vi "main.vi"() -> ()   [LabVIEW 2023] (continued)
     09\t16\t00\t00\tFF\tFF\tB0\t01\r\n       146  18F108A7   00000004    8        F0\t00\t00\tFF\tFF\tFF\tFF\t3E\r\n       145  18F106A7   00000004    8        00\tF7\tFF\tFF\tFF\tFF\tFF\t73\r\n       145  0CF104A7   00000004    8        F0\t60\t22\tFC\tFF\tFF\tFF\t39\r\n       144  0CF103A7   00000004    8        17\t1F\t08\t60\tB1\t1F\t08\t39\r\n       172  1FFFFFFF   00000004    8        00\t00\tFF\tFF\tFF\tFF\tFF\tFF\r\n       163  0CF102A7   00000004    8        30\t75\tE0\t2E\t80\tFF\tFF\tFD\r\n       163  0CF101A7   00000004    8        68\t00\t97\tCC\t00\t15\t39\t22\r\n       162  1FFFFFFF   00000004    8        00\t00\tFF\tFF\tFF\tFF\tFF\tFF\r\n       152  1FFFFFFF   00000004    8        00\t20\tFF\tFF\tFF\tFF\tFF\tFF\r\n       148  1FFFFFFF   00000004    8        00\t00\tFF\tFF\tFF\tFF\tFF\tFF\r\n       147  18FEF117   00000004    8        F7\t97\tCC\tCF\tFF\tFF\tFF\tFF\r\n       147  18F121F0   00000004    8        09\t16\t00\t00\tFF\tFF\tB0\t01\r\n       146  18F108A7   00000004    8        F0\t00\t00\tFF\tFF\tFF\tFF\t3E\r\n       145  18F106A7   00000004    8        00\tF7\tFF\tFF\tFF\tFF\tFF\t73\r\n       145  0CF104A7   00000004    8        F0\t60\t22\tFC\tFF\tFF\tFF\t39\r\n       182  1FFFFFFF   00000004    8        00\t00\tFF\tFF\tFF\tFF\tFF\tFF\r\n       172  1FFFFFFF   00000004    8        00\t00\tFF\tFF\tFF\tFF\tFF\tFF\r\n       163  0CF102A7   00000004    8        30\t75\tE0\t2E\t80\tFF\tFF\tFD\r\n       163  0CF101A7   00000004    8        68\t00\t97\tCC\t00\t15\t39\t22\r\n       162  1FFFFFFF   00000004    8        00\t00\tFF\tFF\tFF\tFF\tFF\tFF\r\n       152  1FFFFFFF   00000004    8        00\t20\tFF\tFF\tFF\tFF\tFF\tFF\r\n       148  1FFFFFFF   00000004    8        00\t00\tFF\tFF\tFF\tFF\tFF\tFF\r\n       147  18FEF117   00000004    8        F7\t97\tCC\tCF\tFF\tFF\tFF\tFF\r\n       147  18F121F0   00000004    8        09\t16\t00\t00\tFF\tFF\tB0\t01\r\n       146  18F108A7   00000004    8        F0\t00\t00\tFF\tFF\tFF\tFF\t3E\r\n       145  18F106A7   00000004    8        00\tF7\tFF\tFF\tFF\tFF\tFF\t73\r\n       183  0CF101A7   00000004    8        68\t00\t97\tCC\t00\t15\t39\t23\r\n       182  1FFFFFFF   00000004    8        00\t00\tFF\tFF\tFF\tFF\tFF\tFF\r\n       172  1FFFFFFF   00000004    8        00\t00\tFF\tFF\tFF\tFF\tFF\tFF\r\n       163  0CF102A7   00000004    8        30\t75\tE0\t2E\t80\tFF\tFF\tFD\r\n       163  0CF101A7   00000004    8        68\t00\t97\tCC\t00\t15\t39\t22\r\n       162  1FFFFFFF   00000004    8        00\t00\tFF\tFF\tFF\tFF\tFF\tFF\r\n       152  1FFFFFFF   00000004    8        00\t20\tFF\tFF\tFF\tFF\tFF\tFF\r\n       148  1FFFFFFF   00000004    8        00\t00\tFF\tFF\tFF\tFF\tFF\tFF\r\n       147  18FEF117   00000004    8        F7\t97\tCC\tCF\tFF\tFF\tFF\tFF\r\n       147  18F121F0   00000004    8        09\t16\t00\t00\tFF\tFF\tB0\t01\r\n       146  18F108A7   00000004    8        F0\t00\t00\tFF\tFF\tFF\tFF\t3E\r\n       183  0CF102A7   00000004    8        30\t75\tE0\t2E\t80\tFF\tFF\tFD\r\n       183  0CF101A7   00000004    8        68\t00\t97\tCC\t00\t15\t39\t23\r\n       182  1FFFFFFF   00000004    8        00\t00\tFF\tFF\tFF\tFF\tFF\tFF\r\n       172  1FFFFFFF   00000004    8        00\t00\tFF\tFF\tFF\tFF\tFF\tFF\r\n       163  0CF102A7   00000004    8        30\t75\tE0\t2E\t80\tFF\tFF\tFD\r\n       163  0CF101A7   00000004    8        68\t00\t97\tCC\t00\t15\t39\t22\r\n       162  1FFFFFFF   00000004    8        00\t00\tFF\tFF\tFF\tFF\tFF\tFF\r\n       152  1FFFFFFF   00000004    8        00\t20\tFF\tFF\tFF\tFF\tFF\tFF\r\n       148  1FFFFFFF   00000004    8        00\t00\tFF\tFF\tFF\tFF\tFF\tFF\r\n       147  18FEF117   00000004    8        F7\t97\tCC\tCF\tFF\tFF\tFF\tFF\r\n       147  18F121F0   00000004    8        09\t16\t00\t00\tFF\tFF\tB0\t01\r\n       192  1FFFFFFF   00000004    8        00\t00\tFF\tFF\tFF\tFF\tFF\tFF\r\n       183  0CF102A7   00000004    8        30\t75\tE0\t2E\t80\tFF\tFF\tFD\r\n       183  0CF101A7   00000004    8        68\t00\t97\tCC\t00\t15\t39\t23\r\n       182  1FFFFFFF   00000004    8        00\t00\tFF\tFF\tFF\tFF\tFF\tFF\r\n       172  1FFFFFFF   00000004    8        00\t00\tFF\tFF\tFF\tFF\tFF\tFF\r\n       163  0CF102A7   00000004    8        30\t75\tE0\t2E\t80\tFF\tFF\tFD\r\n       163  0CF101A7   00000004    8        68\t00\t97\tCC\t00\t15\t39\t22\r\n       162  1FFFFFFF   00000004    8        00\t00\tFF\tFF\tFF\tFF\tFF\tFF\r\n       152  1FFFFFFF   00000004    8        00\t20\tFF\tFF\tFF\tFF\tFF\tFF\r\n       148  1FFFFFFF   00000004    8        00\t00\tFF\tFF\tFF\tFF\tFF\tFF\r\n       147  18FEF117   00000004    8        F7\t97\tCC\tCF\tFF\tFF\tFF\tFF\r\n       193  18F106A7   00000004    8        00\tF7\tFF\tFF\tFF\tFF\tFF\t74\r\n       192  1FFFFFFF   00000004    8        00\t00\tFF\tFF\tFF\tFF\tFF\tFF\r\n       183  0CF102A7   00000004    8        30\t75\tE0\t2E\t80\tFF\tFF\tFD\r\n       183  0CF101A7   00000004    8        68\t00\t97\tCC\t00\t15\t39\t23\r\n       182  1FFFFFFF   00000004    8        00\t00\tFF\tFF\tFF\tFF\tFF\tFF\r\n       172  1FFFFFFF   00000004    8        00\t00\tFF\tFF\tFF\tFF\tFF\tFF\r\n       163  0CF102A7   00000004    8        30\t75\tE0\t2E\t80\tFF\tFF\tFD\r\n       163  0CF101A7   00000004    8        68\t00\t97\tCC\t00\t15\t39\t22\r\n       162  1FFFFFFF   00000004    8        00\t00\tFF\tFF\tFF\tFF\tFF\tFF\r\n       152  1FFFFFFF   00000004    8        00\t20\tFF\tFF\tFF\tFF\tFF\tFF\r\n       148  1FFFFFFF   00000004    8        00\t00\tFF\tFF\tFF\tFF\tFF\tFF\r\n       202  1FFFFFFF   00000004    8        00\t00\tFF\tFF\tFF\tFF\tFF\tFF\r\n       193  18F106A7   00000004    8        00\tF7\tFF\tFF\tFF\tFF\tFF\t74\r\n       192  1FFFFFFF   00000004    8        00\t00\tFF\tFF\tFF\tFF\tFF\tFF\r\n       183  0CF102A7   00000004    8        30\t75\tE0\t2E\t80\tFF\tFF\tFD\r\n       183  0CF101A7   00000004    8        68\t00\t97\tCC\t00\t15\t39\t23\r\n       182  1FFFFFFF   00000004    8        00\t00\tFF\tFF\tFF\tFF\tFF\tFF\r\n       172  1FFFFFFF   00000004    8        00\t00\tFF\tFF\tFF\tFF\tFF\tFF\r\n       163  0CF102A7   00000004    8        30\t75\tE0\t2E\t80\tFF\tFF\tFD\r\n       163  0CF101A7   00000004    8        68\t00\t97\tCC\t00\t15\t39\t22\r\n       162  1FFFFFFF   00000004    8        00\t00\tFF\tFF\tFF\tFF\tFF\tFF\r\n       152  1FFFFFFF   00000004    8        00\t20\tFF\tFF\tFF\tFF\tFF\tFF\r\n       203  0CF101A7   00000004    8        68\t00\t97\tCC\t00\t15\t39\t24\r\n       202  1FFFFFFF   00000004    8        00\t00\tFF\tFF\tFF\tFF\tFF\tFF\r\n       193  18F106A7   00000004    8        00\tF7\tFF\tFF\tFF\tFF\tFF\t74\r\n       192  1FFFFFFF   00000004    8        00\t00\tFF\tFF\tFF\tFF\tFF\tFF\r\n       183  0CF102A7   00000004    8        30\t75\tE0\t2E\t80\tFF\tFF\tFD\r\n       183  0CF101A7   00000004    8        68\t00\t97\tCC\t00\t15\t39\t23\r\n       182  1FFFFFFF   00000004    8        00\t00\tFF\tFF\tFF\tFF\tFF\tFF\r\n       172  1FFFFFFF   00000004    8        00\t00\tFF\tFF\tFF\tFF\tFF\tFF\r\n       163  0CF102A7   00000004    8        30\t75\tE0\t2E\t80\tFF\tFF\tFD\r\n       163  0CF101A7   00000004    8        68\t00\t97\tCC\t00\t15\t39\t22\r\n       162  1FFFFFFF   00000004    8        00\t00\tFF\tFF\tFF\tFF\tFF\tFF\r\n       203  0CF102A7   00000004    8        30\t75\tE0\t2E\t80\tFF\tFF\tFD\r\n       203  0CF101A7   00000004    8        68\t00\t97\tCC\t00\t15\t39\t24\r\n       202  1FFFFFFF   00000004    8        00\t00\tFF\tFF\tFF\tFF\tFF\tFF\r\n       193  18F106A7   00000004    8        00\tF7\tFF\tFF\tFF\tFF\tFF\t74\r\n       192  1FFFFFFF   00000004    8        00\t00\tFF\tFF\tFF\tFF\tFF\tFF\r\n       183  0CF102A7   00000004    8        30\t75\tE0\t2E\t80\tFF\tFF\tFD\r\n       183  0CF101A7   00000004    8        68\t00\t97\tCC\t00\t15\t39\t23\r\n       182  1FFFFFFF   00000004    8        00\t00\tFF\tFF\tFF\tFF\tFF\tFF\r\n       172  1FFFFFFF   00000004    8        00\t00\tFF\tFF\tFF\tFF\tFF\tFF\r\n       163  0CF102A7   00000004    8        30\t75\tE0\t2E\t80\tFF\tFF\tFD\r\n       163  0CF101A7   00000004    8        68\t00\t97\tCC\t00\t15\t39\t22\r\n       212  1FFFFFFF   00000004    8        00\t00\tFF\tFF\tFF\tFF\tFF\tFF\r\n       203  0CF102A7   00000004    8        30\t75\tE0\t2E\t80\tFF\tFF\tFD\r\n       203  0CF101A7   00000004    8        68\t00\t97\tCC\t00\t15\t39\t24\r\n       202  1FFFFFFF   00000004    8        00\t00\tFF\tFF\tFF\tFF\tFF\tFF\r\n       193  18F106A7   00000004    8        00\tF7\tFF\tFF\tFF\tFF\tFF\t74\r\n       192  1FFFFFFF   00000004    8        00\t00\tFF\tFF\tFF\tFF\tFF\tFF\r\n       183  0CF102A7   00000004    8        30\t75\tE0\t2E\t80\tFF\tFF\tFD\r\n       183  0CF101A7   00000004    8        68\t00\t97\tCC\t00\t15\t39\t23\r\n       182  1FFFFFFF   00000004    8        00\t00\tFF\tFF\tFF\tFF\tFF\tFF\r\n       172  1FFFFFFF   00000004    8        00\t00\tFF\tFF\tFF\tFF\tFF\tFF\r\n       163  0CF102A7   00000004    8        30\t75\tE0\t2E\t80\tFF\tFF\tFD\r\n       222  1FFFFFFF   00000004    8        00\t00\tFF\tFF\tFF\tFF\tFF\tFF\r\n       212  1FFFFFFF   00000004    8        00\t00\tFF\tFF\tFF\tFF\tFF\tFF\r\n       203  0CF102A7   00000004    8        30\t75\tE0\t2E\t80\tFF\tFF\tFD\r\n       203  0CF101A7   00000004    8        68\t00\t97\tCC\t00\t15\t39\t24\r\n       202  1FFFFFFF   00000004    8        00\t00\tFF\tFF\tFF\tFF\tFF\tFF\r\n       193  18F106A7   00000004    8        00\tF7\tFF\tFF\tFF\tFF\tFF\t74\r\n       192  1FFFFFFF   00000004    8        00\t00\tFF\tFF\tFF\tFF\tFF\tFF\r\n       183  0CF102A7   00000004    8        30\t75\tE0\t2E\t80\tFF\tFF\tFD\r\n       183  0CF101A7   00000004    8        68\t00\t97\tCC\t00\t15\t39\t23\r\n       182  1FFFFFFF   00000004    8        00\t00\tFF\tFF\tFF\tFF\tFF\tFF\r\n       172  1FFFFFFF   00000004    8        00\t00\tFF\tFF\tFF\tFF\tFF\tFF\r\n       223  0CF101A7   00000004    8        68\t00\t97\tCC\t00\t15\t39\t25\r\n       222  1FFFFFFF   00000004    8        00\t00\tFF\tFF\tFF\tFF\tFF\tFF\r\n       212  1FFFFFFF   00000004    8        00\t00\tFF\tFF\tFF\tFF\tFF\tFF\r\n       203  0CF102A7   00000004    8        30\t75\tE0\t2E\t80\tFF\tFF\tFD\r\n       203  0CF101A7   00000004    8        68\t00\t97\tCC\t00\t15\t39\t24\r\n       202  1FFFFFFF   00000004    8        00\t00\tFF\tFF\tFF\tFF\tFF\tFF\r\n       193  18F106A7   00000004    8        00\tF7\tFF\tFF\tFF\tFF\tFF\t74\r\n       192  1FFFFFFF   00000004    8        00\t00\tFF\tFF\tFF\tFF\tFF\tFF\r\n       183  0CF102A7   00000004    8        30\t75\tE0\t2E\t80\tFF\tFF\tFD\r\n       183  0CF101A7   00000004    8        68\t00\t97\tCC\t00\t15\t39\t23\r\n       182  1FFFFFFF   00000004    8        00\t00\tFF\tFF\tFF\tFF\tFF\tFF\r\n       223  0CF102A7   00000004    8        30\t75\tE0\t2E\t80\tFF\tFF\tFD\r\n       223  0CF101A7   00000004    8        68\t00\t97\tCC\t00\t15\t39\t25\r\n       222  1FFFFFFF   00000004    8        00\t00\tFF\tFF\tFF\tFF\tFF\tFF\r\n       212  1FFFFFFF   00000004    8        00\t00\tFF\tFF\tFF\tFF\tFF\tFF\r\n       203  0CF102A7   00000004    8        30\t75\tE0\t2E\t80\tFF\tFF\tFD\r\n       203  0CF101A7   00000004    8        68\t00\t97\tCC\t00\t15\t39\t24\r\n       202  1FFFFFFF   00000004    8        00\t00\tFF\tFF\tFF\tFF\tFF\tFF\r\n       193  18F106A7   00000004    8        00\tF7\tFF\tFF\tFF\tFF\tFF\t74\r\n       192  1FFFFFFF   00000004    8        00\t00\tFF\tFF\tFF\tFF\tFF\tFF\r\n       183  0CF102A7   00000004    8        30\t75\tE0\t2E\t80\tFF\tFF\tFD\r\n       183  0CF101A7   00000004    8        68\t00\t97\tCC\t00\t15\t39\t23\r\n       232  1FFFFFFF   00000004    8        00\t00\tFF\tFF\tFF\tFF\tFF\tFF\r\n       223  0CF102A7   00000004    8        30\t75\tE0\t2E\t80\tFF\tFF\tFD\r\n       223  0CF101A7   00000004    8        68\t00\t97\tCC\t00\t15\t39\t25\r\n       222  1FFFFFFF   00000004    8        00\t00\tFF\tFF\tFF\tFF\tFF\tFF\r\n       212  1FFFFFFF   00000004    8        00\t00\tFF\tFF\tFF\tFF\tFF\tFF\r\n       203  0CF102A7   00000004    8        30\t75\tE0\t2E\t80\tFF\tFF\tFD\r\n       203  0CF101A7   00000004    8        68\t00\t97\tCC\t00\t15\t39\t24\r\n       202  1FFFFFFF   00000004    8        00\t00\tFF\tFF\tFF\tFF\tFF\tFF\r\n       193  18F106A7   00000004    8        00\tF7\tFF\tFF\tFF\tFF\tFF\t74\r\n       192  1FFFFFFF   00000004    8        00\t00\tFF\tFF\tFF\tFF\tFF\tFF\r\n       183  0CF102A7   00000004    8        30\t75\tE0\t2E\t80\tFF\tFF\tFD\r\n       241  18F11FF0   00000004    8        FF\t3F\t90\t68\t88\t1B\t10\tAC\r\n       232  1FFFFFFF   00000004    8        00\t00\tFF\tFF\tFF\tFF\tFF\tFF\r\n       223  0CF102A7   00000004    8        30\t75\tE0\t2E\t80\tFF\tFF\tFD\r\n       223  0CF101A7   00000004    8        68\t00\t97\tCC\t00\t15\t39\t25\r\n       222  1FFFFFFF   00000004    8        00\t00\tFF\tFF\tFF\tFF\tFF\tFF\r\n       212  1FFFFFFF   00000004    8        00\t00\tFF\tFF\tFF\tFF\tFF\tFF\r\n       203  0CF102A7   00000004    8        30\t75\tE0\t2E\t80\tFF\tFF\tFD\r\n       203  0CF101A7   00000004    8        68\t00\t97\tCC\t00\t15\t39\t24\r\n       202  1FFFFFFF   00000004    8        00\t00\tFF\tFF\tFF\tFF\tFF\tFF\r\n       193  18F106A7   00000004    8        00\tF7\tFF\tFF\tFF\tFF\tFF\t74\r\n       192  1FFFFFFF   00000004    8        00\t00\tFF\tFF\tFF\tFF\tFF\tFF\r\n       242  18F120F0   00000004    8        2B\t75\t60\tB1\tB0\t01\tFF\tFF\r\n       241  18F11FF0   00000004    8        FF\t3F\t90\t68\t88\t1B\t10\tAC\r\n       232  1FFFFFFF   00000004    8        00\t00\tFF\tFF\tFF\tFF\tFF\tFF\r\n       223  0CF102A7   00000004    8        30\t75\tE0\t2E\t80\tFF\tFF\tFD\r\n       223  0CF101A7   00000004    8        68\t00\t97\tCC\t00\t15\t39\t25\r\n       222  1FFFFFFF   00000004    8        00\t00\tFF\tFF\tFF\tFF\tFF\tFF\r\n       212  1FFFFFFF   00000004    8        00\t00\tFF\tFF\tFF\tFF\tFF\tFF\r\n       203  0CF102A7   00000004    8        30\t75\tE0\t2E\t80\tFF\tFF\tFD\r\n       203  0CF101A7   00000004    8        68\t00\t97\tCC\t00\t15\t39\t24\r\n       202  1FFFFFFF   00000004    8        00\t00\tFF\tFF\tFF\tFF\tFF\tFF\r\n       193  18F106A7   00000004    8        00\tF7\tFF\tFF\tFF\tFF\tFF\t74\r\n       243  0CF101A7   00000004    8        68\t00\t97\tCC\t00\t15\t39\t26\r\n       242  18F120F0   00000004    8        2B\t75\t60\tB1\tB0\t01\tFF\tFF\r\n       241  18F11FF0   00000004    8        FF\t3F\t90\t68\t88\t1B\t10\tAC\r\n       232  1FFFFFFF   00000004    8        00\t00\tFF\tFF\tFF\tFF\tFF\tFF\r\n       223  0CF102A7   00000004    8        30\t75\tE0\t2E\t80\tFF\tFF\tFD\r\n       223  0CF101A7   00000004    8        68\t00\t97\tCC\t00\t15\t39\t25\r\n       222  1FFFFFFF   00000004    8        00\t00\tFF\tFF\tFF\tFF\tFF\tFF\r\n       212  1FFFFFFF   00000004    8        00\t00\tFF\tFF\tFF\tFF\tFF\tFF\r\n       203  0CF102A7   00000004    8        30\t75\tE0\t2E\t80\tFF\tFF\tFD\r\n       203  0CF101A7   00000004    8        68\t00\t97\tCC\t00\t15\t39\t24\r\n       202  1FFFFFFF   00000004    8        00\t00\tFF\tFF\tFF\tFF\tFF\tFF\r\n       243  0C3C4D4A   00000004    8        BE\tFF\tFF\t7F\t18\tFF\tFF\t3A\r\n       243  0CF101A7   00000004    8        68\t00\t97\tCC\t00\t15\t39\t26\r\n       242  18F120F0   00000004    8        2B\t75\t60\tB1\tB0\t01\tFF\tFF\r\n       241  18F11FF0   00000004    8        FF\t3F\t90\t68\t88\t1B\t10\tAC\r\n       232  1FFFFFFF   00000004    8        00\t00\tFF\tFF\tFF\tFF\tFF\tFF\r\n       223  0CF102A7   00000004    8        30\t75\tE0\t2E\t80\tFF\tFF\tFD\r\n       223  0CF101A7   00000004    8        68\t00\t97\tCC\t00\t15\t39\t25\r\n       222  1FFFFFFF   00000004    8        00\t00\tFF\tFF\tFF\tFF\tFF\tFF\r\n       212  1FFFFFFF   00000004    8        00\t00\tFF\tFF\tFF\tFF\tFF\tFF\r\n       203  0CF102A7   00000004    8        30\t75\tE0\t2E\t80\tFF\tFF\tFD\r\n       203  0CF101A7   00000004    8        68\t00\t97\tCC\t00\t15\t39\t24\r\n       244  0CF102A7   00000004    8        30\t75\tE0\t2E\t80\tFF\tFF\tFD\r\n       243  0C3C4D4A   00000004    8        BE\tFF\tFF\t7F\t18\tFF\tFF\t3A\r\n       243  0CF101A7   00000004    8        68\t00\t97\tCC\t00\t15\t39\t26\r\n       242  18F120F0   00000004    8        2B\t75\t60\tB1\tB0\t01\tFF\tFF\r\n       241  18F11FF0   00000004    8        FF\t3F\t90\t68\t88\t1B\t10\tAC\r\n       232  1FFFFFFF   00000004    8        00\t00\tFF\tFF\tFF\tFF\tFF\tFF\r\n       223  0CF102A7   00000004    8        30\t75\tE0\t2E\t80\tFF\tFF\tFD\r\n       223  0CF101A7   00000004    8        68\t00\t97\tCC\t00\t15\t39\t25\r\n       222  1FFFFFFF   00000004    8        00\t00\tFF\tFF\tFF\tFF\tFF\tFF\r\n       212  1FFFFFFF   00000004    8        00\t00\tFF\tFF\tFF\tFF\tFF\tFF\r\n       203  0CF102A7   00000004    8        30\t75\tE0\t2E\t80\tFF\tFF\tFD\r\n       244  0CF103A7   00000004    8        17\t1F\t08\t60\tB1\t1F\t08\t3A\r\n       244  0CF102A7   00000004    8        30\t75\tE0\t2E\t80\tFF\tFF\tFD\r\n       243  0C3C4D4A   00000004    8        BE\tFF\tFF\t7F\t18\tFF\tFF\t3A\r\n       243  0CF101A7   00000004    8        68\t00\t97\tCC\t00\t15\t39\t26\r\n       242  18F120F0   00000004    8        2B\t75\t60\tB1\tB0\t01\tFF\tFF\r\n       241  18F11FF0   00000004    8        FF\t3F\t90\t68\t88\t1B\t10\tAC\r\n       232  1FFFFFFF   00000004    8        00\t00\tFF\tFF\tFF\tFF\tFF\tFF\r\n       223  0CF102A7   00000004    8        30\t75\tE0\t2E\t80\tFF\tFF\tFD\r\n       223  0CF101A7   00000004    8        68\t00\t97\tCC\t00\t15\t39\t25\r\n       222  1FFFFFFF   00000004    8        00\t00\tFF\tFF\tFF\tFF\tFF\tFF\r\n       212  1FFFFFFF   00000004    8        00\t00\tFF\tFF\tFF\tFF\tFF\tFF\r\n       245  0CF104A7   00000004    8        F0\t60\t22\tFC\tFF\tFF\tFF\t3A\r\n       244  0CF103A7   00000004    8        17\t1F\t08\t60\tB1\t1F\t08\t3A\r\n       244  0CF102A7   00000004    8        30\t75\tE0\t2E\t80\tFF\tFF\tFD\r\n       243  0C3C4D4A   00000004    8        BE\tFF\tFF\t7F\t18\tFF\tFF\t3A\r\n       243  0CF101A7   00000004    8        68\t00\t97\tCC\t00\t15\t39\t26\r\n       242  18F120F0   00000004    8        2B\t75\t60\tB1\tB0\t01\tFF\tFF\r\n       241  18F11FF0   00000004    8        FF\t3F\t90\t68\t88\t1B\t10\tAC\r\n       232  1FFFFFFF   00000004    8        00\t00\tFF\tFF\tFF\tFF\tFF\tFF\r\n       223  0CF102A7   00000004    8        30\t75\tE0\t2E\t80\tFF\tFF\tFD\r\n       223  0CF101A7   00000004    8        68\t00\t97\tCC\t00\t15\t39\t25\r\n       222  1FFFFFFF   00000004    8        00\t00\tFF\tFF\tFF\tFF\tFF\tFF\r\n       246  18F106A7   00000004    8        00\tF7\tFF\tFF\tFF\tFF\tFF\t75\r\n       245  0CF104A7   00000004    8        F0\t60\t22\tFC\tFF\tFF\tFF\t3A\r\n       244  0CF103A7   00000004    8        17\t1F\t08\t60\tB1\t1F\t08\t3A\r\n       244  0CF102A7   00000004    8        30\t75\tE0\t2E\t80\tFF\tFF\tFD\r\n       243  0C3C4D4A   00000004    8        BE\tFF\tFF\t7F\t18\tFF\tFF\t3A\r\n       243  0CF101A7   00000004    8        68\t00\t97\tCC\t00\t15\t39\t26\r\n       242  18F120F0   00000004    8        2B\t75\t60\tB1\tB0\t01\tFF\tFF\r\n       241  18F11FF0   00000004    8        FF\t3F\t90\t68\t88\t1B\t10\tAC\r\n       232  1FFFFFFF   00000004    8        00\t00\tFF\tFF\tFF\tFF\tFF\tFF\r\n       223  0CF102A7   00000004    8        30\t75\tE0\t2E\t80\tFF\tFF\tFD\r\n       223  0CF101A7   00000004    8        68\t00\t97\tCC\t00\t15\t39\t25\r\n       246  18F121F0   00000004    8        09\t16\t00\t00\tFF\tFF\tB0\t01\r\n       246  18F106A7   00000004    8        00\tF7\tFF\tFF\tFF\tFF\tFF\t75\r\n       245  0CF104A7   00000004    8        F0\t60\t22\tFC\tFF\tFF\tFF\t3A\r\n       244  0CF103A7   00000004    8        17\t1F\t08\t60\tB1\t1F\t08\t3A\r\n       244  0CF102A7   00000004    8        30\t75\tE0\t2E\t80\tFF\tFF\tFD\r\n       243  0C3C4D4A   00000004    8        BE\tFF\tFF\t7F\t18\tFF\tFF\t3A\r\n       243  0CF101A7   00000004    8        68\t00\t97\tCC\t00\t15\t39\t26\r\n       242  18F120F0   00000004    8        2B\t75\t60\tB1\tB0\t01\tFF\tFF\r\n       241  18F11FF0   00000004    8        FF\t3F\t90\t68\t88\t1B\t10\tAC\r\n       232  1FFFFFFF   00000004    8        00\t00\tFF\tFF\tFF\tFF\tFF\tFF\r\n       223  0CF102A7   00000004    8        30\t75\tE0\t2E\t80\tFF\tFF\tFD\r\n       247  1FFFFFFF   00000004    8        00\t00\tFF\tFF\tFF\tFF\tFF\tFF\r\n       246  18F121F0   00000004    8        09\t16\t00\t00\tFF\tFF\tB0\t01\r\n       246  18F106A7   00000004    8        00\tF7\tFF\tFF\tFF\tFF\tFF\t75\r\n       245  0CF104A7   00000004    8        F0\t60\t22\tFC\tFF\tFF\tFF\t3A\r\n       244  0CF103A7   00000004    8        17\t1F\t08\t60\tB1\t1F\t08\t3A\r\n       244  0CF102A7   00000004    8        30\t75\tE0\t2E\t80\tFF\tFF\tFD\r\n       243  0C3C4D4A   00000004    8        BE\tFF\tFF\t7F\t18\tFF\tFF\t3A\r\n       243  0CF101A7   00000004    8        68\t00\t97\tCC\t00\t15\t39\t26\r\n       242  18F120F0   00000004    8        2B\t75\t60\tB1\tB0\t01\tFF\tFF\r\n       241  18F11FF0   00000004    8        FF\t3F\t90\t68\t88\t1B\t10\tAC\r\n       232  1FFFFFFF   00000004    8        00\t00\tFF\tFF\tFF\tFF\tFF\tFF\r\n       252  1FFFFFFF   00000004    8        00\t00\tFF\tFF\tFF\tFF\tFF\tFF\r\n       247  1FFFFFFF   00000004    8        00\t00\tFF\tFF\tFF\tFF\tFF\tFF\r\n       246  18F121F0   00000004    8        09\t16\t00\t00\tFF\tFF\tB0\t01\r\n       246  18F106A7   00000004    8        00\tF7\tFF\tFF\tFF\tFF\tFF\t75\r\n       245  0CF104A7   00000004    8        F0\t60\t22\tFC\tFF\tFF\tFF\t3A\r\n       244  0CF103A7   00000004    8        17\t1F\t08\t60\tB1\t1F\t08\t3A\r\n       244  0CF102A7   00000004    8        30\t75\tE0\t2E\t80\tFF\tFF\tFD\r\n       243  0C3C4D4A   00000004    8        BE\tFF\tFF\t7F\t18\tFF\tFF\t3A\r\n       243  0CF101A7   00000004    8        68\t00\t97\tCC\t00\t15\t39\t26\r\n       242  18F120F0   00000004    8        2B\t75\t60\tB1\tB0\t01\tFF\tFF\r\n       241  18F11FF0   00000004    8        FF\t3F\t90\t68\t88\t1B\t10\tAC\r\n       262  1FFFFFFF   00000004    8        00\t20\tFF\tFF\tFF\tFF\tFF\tFF\r\n       252  1FFFFFFF   00000004    8        00\t00\tFF\tFF\tFF\tFF\tFF\tFF\r\n       247  1FFFFFFF   00000004    8        00\t00\tFF\tFF\tFF\tFF\tFF\tFF\r\n       246  18F121F0   00000004    8        09\t16\t00\t00\tFF\tFF\tB0\t01\r\n       246  18F106A7   00000004    8        00\tF7\tFF\tFF\tFF\tFF\tFF\t75\r\n       245  0CF104A7   00000004    8        F0\t60\t22\tFC\tFF\tFF\tFF\t3A\r\n       244  0CF103A7   00000004    8        17\t1F\t08\t60\tB1\t1F\t08\t3A\r\n       244  0CF102A7   00000004    8        30\t75\tE0\t2E\t80\tFF\tFF\tFD\r\n       243  0C3C4D4A   00000004    8        BE\tFF\tFF\t7F\t18\tFF\tFF\t3A\r\n       243  0CF101A7   00000004    8        68\t00\t97\tCC\t00\t15\t39\t26\r\n       242  18F120F0   00000004    8        2B\t75\t60\tB1\tB0\t01\tFF\tFF\r\n       263  0CF101A7   00000004    8        68\t00\t97\tCC\t00\t15\t39\t27\r\n       262  1FFFFFFF   00000004    8        00\t20\tFF\tFF\tFF\tFF\tFF\tFF\r\n       252  1FFFFFFF   00000004    8        00\t00\tFF\tFF\tFF\tFF\tFF\tFF\r\n       247  1FFFFFFF   00000004    8        00\t00\tFF\tFF\tFF\tFF\tFF\tFF\r\n       246  18F121F0   00000004    8        09\t16\t00\t00\tFF\tFF\tB0\t01\r\n       246  18F106A7   00000004    8        00\tF7\tFF\tFF\tFF\tFF\tFF\t75\r\n       245  0CF104A7   00000004    8        F0\t60\t22\tFC\tFF\tFF\tFF\t3A\r\n       244  0CF103A7   00000004    8        17\t1F\t08\t60\tB1\t1F\t08\t3A\r\n       244  0CF102A7   00000004    8        30\t75\tE0\t2E\t80\tFF\tFF\tFD\r\n       243  0C3C4D4A   00000004    8        BE\tFF\tFF\t7F\t18\tFF\tFF\t3A\r\n       243  0CF101A7   00000004    8        68\t00\t97\tCC\t00\t15\t39\t26\r\n       263  0CF102A7   00000004    8        30\t75\tE0\t2E\t80\tFF\tFF\tFD\r\n       263  0CF101A7   00000004    8        68\t00\t97\tCC\t00\t15\t39\t27\r\n       262  1FFFFFFF   00000004    8        00\t20\tFF\tFF\tFF\tFF\tFF\tFF\r\n       252  1FFFFFFF   00000004    8        00\t00\tFF\tFF\tFF\tFF\tFF\tFF\r\n       247  1FFFFFFF   00000004    8        00\t00\tFF\tFF\tFF\tFF\tFF\tFF\r\n       246  18F121F0   00000004    8        09\t16\t00\t00\tFF\tFF\tB0\t01\r\n       246  18F106A7   00000004    8        00\tF7\tFF\tFF\tFF\tFF\tFF\t75\r\n       245  0CF104A7   00000004    8        F0\t60\t22\tFC\tFF\tFF\tFF\t3A\r\n       244  0CF103A7   00000004    8        17\t1F\t08\t60\tB1\t1F\t08\t3A\r\n       244  0CF102A7   00000004    8        30\t75\tE0\t2E\t80\tFF\tFF\tFD\r\n       243  0C3C4D4A   00000004    8        BE\tFF\tFF\t7F\t18\tFF\tFF\t3A\r\n       272  1FFFFFFF   00000004    8        00\t00\tFF\tFF\tFF\tFF\tFF\tFF\r\n       263  0CF102A7   00000004    8        30\t75\tE0\t2E\t80\tFF\tFF\tFD\r\n       263  0CF101A7   00000004    8        68\t00\t97\tCC\t00\t15\t39\t27\r\n       262  1FFFFFFF   00000004    8        00\t20\tFF\tFF\tFF\tFF\tFF\tFF\r\n       252  1FFFFFFF   00000004    8        00\t00\tFF\tFF\tFF\tFF\tFF\tFF\r\n       247  1FFFFFFF   00000004    8        00\t00\tFF\tFF\tFF\tFF\tFF\tFF\r\n       246  18F121F0   00000004    8        09\t16\t00\t00\tFF\tFF\tB0\t01\r\n       246  18F106A7   00000004    8        00\tF7\tFF\tFF\tFF\tFF\tFF\t75\r\n       245  0CF104A7   00000004    8        F0\t60\t22\tFC\tFF\tFF\tFF\t3A\r\n       244  0CF103A7   00000004    8        17\t1F\t08\t60\tB1\t1F\t08\t3A\r\n       244  0CF102A7   00000004    8        30\t75\tE0\t2E\t80\tFF\tFF\tFD\r\n       282  1FFFFFFF   00000004    8        00\t00\tFF\tFF\tFF\tFF\tFF\tFF\r\n       272  1FFFFFFF   00000004    8        00\t00\tFF\tFF\tFF\tFF\tFF\tFF\r\n       263  0CF102A7   00000004    8        30\t75\tE0\t2E\t80\tFF\tFF\tFD\r\n       263  0CF101A7   00000004    8        68\t00\t97\tCC\t00\t15\t39\t27\r\n       262  1FFFFFFF   00000004    8        00\t20\tFF\tFF\tFF\tFF\tFF\tFF\r\n       252  1FFFFFFF   00000004    8        00\t00\tFF\tFF\tFF\tFF\tFF\tFF\r\n       247  1FFFFFFF   00000004    8        00\t00\tFF\tFF\tFF\tFF\tFF\tFF\r\n       246  18F121F0   00000004    8        09\t16\t00\t00\tFF\tFF\tB0\t01\r\n       246  18F106A7   00000004    8        00\tF7\tFF\tFF\tFF\tFF\tFF\t75\r\n       245  0CF104A7   00000004    8        F0\t60\t22\tFC\tFF\tFF\tFF\t3A\r\n       244  0CF103A7   00000004    8        17\t1F\t08\t60\tB1\t1F\t08\t3A\r\n       283  0CF101A7   00000004    8        68\t00\t97\tCC\t00\t15\t39\t28\r\n       282  1FFFFFFF   00000004    8        00\t00\tFF\tFF\tFF\tFF\tFF\tFF\r\n       272  1FFFFFFF   00000004    8        00\t00\tFF\tFF\tFF\tFF\tFF\tFF\r\n       263  0CF102A7   00000004    8        30\t75\tE0\t2E\t80\tFF\tFF\tFD\r\n       263  0CF101A7   00000004    8        68\t00\t97\tCC\t00\t15\t39\t27\r\n       262  1FFFFFFF   00000004    8        00\t20\tFF\tFF\tFF\tFF\tFF\tFF\r\n       252  1FFFFFFF   00000004    8        00\t00\tFF\tFF\tFF\tFF\tFF\tFF\r\n       247  1FFFFFFF   00000004    8        00\t00\tFF\tFF\tFF\tFF\tFF\tFF\r\n       246  18F121F0   00000004    8        09\t16\t00\t00\tFF\tFF\tB0\t01\r\n       246  18F106A7   00000004    8        00\tF7\tFF\tFF\tFF\tFF\tFF\t75\r\n       245  0CF104A7   00000004    8        F0\t60\t22\tFC\tFF\tFF\tFF\t3A\r\n       283  0CF102A7   00000004    8        30\t75\tE0\t2E\t80\tFF\tFF\tFD\r\n       283  0CF101A7   00000004    8        68\t00\t97\tCC\t00\t15\t39\t28\r\n       282  1FFFFFFF   00000004    8        00\t00\tFF\tFF\tFF\tFF\tFF\tFF\r\n       272  1FFFFFFF   00000004    8        00\t00\tFF\tFF\tFF\tFF\tFF\tFF\r\n       263  0CF102A7   00000004    8        30\t75\tE0\t2E\t80\tFF\tFF\tFD\r\n       263  0CF101A7   00000004    8        68\t00\t97\tCC\t00\t15\t39\t27\r\n       262  1FFFFFFF   00000004    8        00\t20\tFF\tFF\tFF\tFF\tFF\tFF\r\n       252  1FFFFFFF   00000004    8        00\t00\tFF\tFF\tFF\tFF\tFF\tFF\r\n       247  1FFFFFFF   00000004    8        00\t00\tFF\tFF\tFF\tFF\tFF\tFF\r\n       246  18F121F0   00000004    8        09\t16\t00\t00\tFF\tFF\tB0\t01\r\n       246  18F106A7   00000004    8        00\tF7\tFF\tFF\tFF\tFF\tFF\t75\r\n       292  1FFFFFFF   00000004    8        00\t00\tFF\tFF\tFF\tFF\tFF\tFF\r\n       283  0CF102A7   00000004    8        30\t75\tE0\t2E\t80\tFF\tFF\tFD\r\n       283  0CF101A7   00000004    8        68\t00\t97\tCC\t00\t15\t39\t28\r\n       282  1FFFFFFF   00000004    8        00\t00\tFF\tFF\tFF\tFF\tFF\tFF\r\n       272  1FFFFFFF   00000004    8        00\t00\tFF\tFF\tFF\tFF\tFF\tFF\r\n       263  0CF102A7   00000004    8        30\t75\tE0\t2E\t80\tFF\tFF\tFD\r\n       263  0CF101A7   00000004    8        68\t00\t97\tCC\t00\t15\t39\t27\r\n       262  1FFFFFFF   00000004    8        00\t20\tFF\tFF\tFF\tFF\tFF\tFF\r\n       252  1FFFFFFF   00000004    8        00\t00\tFF\tFF\tFF\tFF\tFF\tFF\r\n       247  1FFFFFFF   00000004    8        00\t00\tFF\tFF\tFF\tFF\tFF\tFF\r\n       246  18F121F0   00000004    8        09\t16\t00\t00\tFF\tFF\tB0\t01\r\n       293  18F106A7   00000004    8        00\tF7\tFF\tFF\tFF\tFF\tFF\t76\r\n       292  1FFFFFFF   00000004    8        00\t00\tFF\tFF\tFF\tFF\tFF\tFF\r\n       283  0CF102A7   00000004    8        30\t75\tE0\t2E\t80\tFF\tFF\tFD\r\n       283  0CF101A7   00000004    8        68\t00\t97\tCC\t00\t15\t39\t28\r\n       282  1FFFFFFF   00000004    8        00\t00\tFF\tFF\tFF\tFF\tFF\tFF\r\n       272  1FFFFFFF   00000004    8        00\t00\tFF\tFF\tFF\tFF\tFF\tFF\r\n       263  0CF102A7   00000004    8        30\t75\tE0\t2E\t80\tFF\tFF\tFD\r\n       263  0CF101A7   00000004    8        68\t00\t97\tCC\t00\t15\t39\t27\r\n       262  1FFFFFFF   00000004    8        00\t20\tFF\tFF\tFF\tFF\tFF\tFF\r\n       252  1FFFFFFF   00000004    8        00\t00\tFF\tFF\tFF\tFF\tFF\tFF\r\n       247  1FFFFFFF   00000004    8        00\t00\tFF\tFF\tFF\tFF\tFF\tFF\r\n       302  1FFFFFFF   00000004    8        00\t00\tFF\tFF\tFF\tFF\tFF\tFF\r\n       293  18F106A7   00000004    8        00\tF7\tFF\tFF\tFF\tFF\tFF\t76\r\n       292  1FFFFFFF   00000004    8        00\t00\tFF\tFF\tFF\tFF\tFF\tFF\r\n       283  0CF102A7   00000004    8        30\t75\tE0\t2E\t80\tFF\tFF\tFD\r\n       283  0CF101A7   00000004    8        68\t00\t97\tCC\t00\t15\t39\t28\r\n       282  1FFFFFFF   00000004    8        00\t00\tFF\tFF\tFF\tFF\tFF\tFF\r\n       272  1FFFFFFF   00000004    8        00\t00\tFF\tFF\tFF\tFF\tFF\tFF\r\n       263  0CF102A7   00000004    8        30\t75\tE0\t2E\t80\tFF\tFF\tFD\r\n       263  0CF101A7   00000004    8        68\t00\t97\tCC\t00\t15\t39\t27\r\n       262  1FFFFFFF   00000004    8        00\t20\tFF\tFF\tFF\tFF\tFF\tFF\r\n       252  1FFFFFFF   00000004    8        00\t00\tFF\tFF\tFF\tFF\tFF\tFF\r\n       303  0CF101A7   00000004    8        68\t00\t97\tCC\t00\t15\t39\t29\r\n       302  1FFFFFFF   00000004    8        00\t00\tFF\tFF\tFF\tFF\tFF\tFF\r\n       293  18F106A7   00000004    8        00\tF7\tFF\tFF\tFF\tFF\tFF\t76\r\n       292  1FFFFFFF   00000004    8        00\t00\tFF\tFF\tFF\tFF\tFF\tFF\r\n       283  0CF102A7   00000004    8        30\t75\tE0\t2E\t80\tFF\tFF\tFD\r\n       283  0CF101A7   00000004    8        68\t00\t97\tCC\t00\t15\t39\t28\r\n       282  1FFFFFFF   00000004    8        00\t00\tFF\tFF\tFF\tFF\tFF\tFF\r\n       272  1FFFFFFF   00000004    8        00\t00\tFF\tFF\tFF\tFF\tFF\tFF\r\n       263  0CF102A7   00000004    8        30\t75\tE0\t2E\t80\tFF\tFF\tFD\r\n       263  0CF101A7   00000004    8        68\t00\t97\tCC\t00\t15\t39\t27\r\n       262  1FFFFFFF   00000004    8        00\t20\tFF\tFF\tFF\tFF\tFF\tFF\r\n       303  0CF102A7   00000004    8        30\t75\tE0\t2E\t80\tFF\tFF\tFD\r\n       303  0CF101A7   00000004    8        68\t00\t97\tCC\t00\t15\t39\t29\r\n       302  1FFFFFFF   00000004    8        00\t00\tFF\tFF\tFF\tFF\tFF\tFF\r\n       293  18F106A7   00000004    8        00\tF7\tFF\tFF\tFF\tFF\tFF\t76\r\n       292  1FFFFFFF   00000004    8        00\t00\tFF\tFF\tFF\tFF\tFF\tFF\r\n       283  0CF102A7   00000004    8        30\t75\tE0\t2E\t80\tFF\tFF\tFD\r\n       283  0CF101A7   00000004    8        68\t00\t97\tCC\t00\t15\t39\t28\r\n       282  1FFFFFFF   00000004    8        00\t00\tFF\tFF\tFF\tFF\tFF\tFF\r\n       272  1FFFFFFF   00000004    8        00\t00\tFF\tFF\tFF\tFF\tFF\tFF\r\n       263  0CF102A7   00000004    8        30\t75\tE0\t2E\t80\tFF\tFF\tFD\r\n       263  0CF101A7   00000004    8        68\t00\t97\tCC\t00\t15\t39\t27\r\n       312  1FFFFFFF   00000004    8        00\t20\tFF\tFF\tFF\tFF\tFF\tFF\r\n       303  0CF102A7   00000004    8        30\t75\tE0\t2E\t80\tFF\tFF\tFD\r\n       303  0CF101A7   00000004    8        68\t00\t97\tCC\t00\t15\t39\t29\r\n       302  1FFFFFFF   00000004    8        00\t00\tFF\tFF\tFF\tFF\tFF\tFF\r\n       293  18F106A7   00000004    8        00\tF7\tFF\tFF\tFF\tFF\tFF\t76\r\n       292  1FFFFFFF   00000004    8        00\t00\tFF\tFF\tFF\tFF\tFF\tFF\r\n       283  0CF102A7   00000004    8        30\t75\tE0\t2E\t80\tFF\tFF\tFD\r\n       283  0CF101A7   00000004    8        68\t00\t97\tCC\t00\t15\t39\t28\r\n       282  1FFFFFFF   00000004    8        00\t00\tFF\tFF\tFF\tFF\tFF\tFF\r\n       272  1FFFFFFF   00000004    8        00\t00\tFF\tFF\tFF\tFF\tFF\tFF\r\n       263  0CF102A7   00000004    8        30\t75\tE0\t2E\t80\tFF\tFF\tFD\r\n       322  1FFFFFFF   00000004    8        00\t20\tFF\tFF\tFF\tFF\tFF\tFF\r\n       312  1FFFFFFF   00000004    8        00\t20\tFF\tFF\tFF\tFF\tFF\tFF\r\n       303  0CF102A7   00000004    8        30\t75\tE0\t2E\t80\tFF\tFF\tFD\r\n       303  0CF101A7   00000004    8        68\t00\t97\tCC\t00\t15\t39\t29\r\n       302  1FFFFFFF   00000004    8        00\t00\tFF\tFF\tFF\tFF\tFF\tFF\r\n       293  18F106A7   00000004    8        00\tF7\tFF\tFF\tFF\tFF\tFF\t76\r\n       292  1FFFFFFF   00000004    8        00\t00\tFF\tFF\tFF\tFF\tFF\tFF\r\n       283  0CF102A7   00000004    8        30\t75\tE0\t2E\t80\tFF\tFF\tFD\r\n       283  0CF101A7   00000004    8        68\t00\t97\tCC\t00\t15\t39\t28\r\n       282  1FFFFFFF   00000004    8        00\t00\tFF\tFF\tFF\tFF\tFF\tFF\r\n       272  1FFFFFFF   00000004    8        00\t00\tFF\tFF\tFF\tFF\tFF\tFF\r\n       323  0CF101A7   00000004    8        68\t00\t97\tCC\t00\t15\t39\t2A\r\n       322  1FFFFFFF   00000004    8        00\t20\tFF\tFF\tFF\tFF\tFF\tFF\r\n       312  1FFFFFFF   00000004    8        00\t20\tFF\tFF\tFF\tFF\tFF\tFF\r\n       303  0CF102A7   00000004    8        30\t75\tE0\t2E\t80\tFF\tFF\tFD\r\n       303  0CF101A7   00000004    8        68\t00\t97\tCC\t00\t15\t39\t29\r\n       302  1FFFFFFF   00000004    8        00\t00\tFF\tFF\tFF\tFF\tFF\tFF\r\n       293  18F106A7   00000004    8        00\tF7\tFF\tFF\tFF\tFF\tFF\t76\r\n       292  1FFFFFFF   00000004    8        00\t00\tFF\tFF\tFF\tFF\tFF\tFF\r\n       283  0CF102A7   00000004    8        30\t75\tE0\t2E\t80\tFF\tFF\tFD\r\n       283  0CF101A7   00000004    8        68\t00\t97\tCC\t00\t15\t39\t28\r\n       282  1FFFFFFF   00000004    8        00\t00\tFF\tFF\tFF\tFF\tFF\tFF\r\n       323  0CF102A7   00000004    8        30\t75\tE0\t2E\t80\tFF\tFF\tFD\r\n       323  0CF101A7   00000004    8        68\t00\t97\tCC\t00\t15\t39\t2A\r\n       322  1FFFFFFF   00000004    8        00\t20\tFF\tFF\tFF\tFF\tFF\tFF\r\n       312  1FFFFFFF   00000004    8        00\t20\tFF\tFF\tFF\tFF\tFF\tFF\r\n       303  0CF102A7   00000004    8        30\t75\tE0\t2E\t80\tFF\tFF\tFD\r\n       303  0CF101A7   00000004    8        68\t00\t97\tCC\t00\t15\t39\t29\r\n       302  1FFFFFFF   00000004    8        00\t00\tFF\tFF\tFF\tFF\tFF\tFF\r\n       293  18F106A7   00000004    8        00\tF7\tFF\tFF\tFF\tFF\tFF\t76\r\n       292  1FFFFFFF   00000004    8        00\t00\tFF\tFF\tFF\tFF\tFF\tFF\r\n       283  0CF102A7   00000004    8        30\t75\tE0\t2E\t80\tFF\tFF\tFD\r\n       283  0CF101A7   00000004    8        68\t00\t97\tCC\t00\t15\t39\t28\r\n       332  1FFFFFFF   00000004    8        00\t00\tFF\tFF\tFF\tFF\tFF\tFF\r\n       323  0CF102A7   00000004    8        30\t75\tE0\t2E\t80\tFF\tFF\tFD\r\n       323  0CF101A7   00000004    8        68\t00\t97\tCC\t00\t15\t39\t2A\r\n       322  1FFFFFFF   00000004    8        00\t20\tFF\tFF\tFF\tFF\tFF\tFF\r\n       312  1FFFFFFF   00000004    8        00\t20\tFF\tFF\tFF\tFF\tFF\tFF\r\n       303  0CF102A7   00000004    8        30\t75\tE0\t2E\t80\tFF\tFF\tFD\r\n       303  0CF101A7   00000004    8        68\t00\t97\tCC\t00\t15\t39\t29\r\n       302  1FFFFFFF   00000004    8        00\t00\tFF\tFF\tFF\tFF\tFF\tFF\r\n       293  18F106A7   00000004    8        00\tF7\tFF\tFF\tFF\tFF\tFF\t76\r\n       292  1FFFFFFF   00000004    8        00\t00\tFF\tFF\tFF\tFF\tFF\tFF\r\n       283  0CF102A7   00000004    8        30\t75\tE0\t2E\t80\tFF\tFF\tFD\r\n       341  18F11FF0   00000004    8        FF\t3F\t90\t68\t88\t1B\t10\tBC\r\n       332  1FFFFFFF   00000004    8        00\t00\tFF\tFF\tFF\tFF\tFF\tFF\r\n       323  0CF102A7   00000004    8        30\t75\tE0\t2E\t80\tFF\tFF\tFD\r\n       323  0CF101A7   00000004    8        68\t00\t97\tCC\t00\t15\t39\t2A\r\n       322  1FFFFFFF   00000004    8        00\t20\tFF\tFF\tFF\tFF\tFF\tFF\r\n       312  1FFFFFFF   00000004    8        00\t20\tFF\tFF\tFF\tFF\tFF\tFF\r\n       303  0CF102A7   00000004    8        30\t75\tE0\t2E\t80\tFF\tFF\tFD\r\n       303  0CF101A7   00000004    8        68\t00\t97\tCC\t00\t15\t39\t29\r\n       302  1FFFFFFF   00000004    8        00\t00\tFF\tFF\tFF\tFF\tFF\tFF\r\n       293  18F106A7   00000004    8        00\tF7\tFF\tFF\tFF\tFF\tFF\t76\r\n       292  1FFFFFFF   00000004    8        00\t00\tFF\tFF\tFF\tFF\tFF\tFF\r\n       342  18F120F0   00000004    8        2B\t75\t60\tB1\tB0\t01\tFF\tFF\r\n       341  18F11FF0   00000004    8        FF\t3F\t90\t68\t88\t1B\t10\tBC\r\n       332  1FFFFFFF   00000004    8        00\t00\tFF\tFF\tFF\tFF\tFF\tFF\r\n       323  0CF102A7   00000004    8        30\t75\tE0\t2E\t80\tFF\tFF\tFD\r\n       323  0CF101A7   00000004    8        68\t00\t97\tCC\t00\t15\t39\t2A\r\n       322  1FFFFFFF   00000004    8        00\t20\tFF\tFF\tFF\tFF\tFF\tFF\r\n       312  1FFFFFFF   00000004    8        00\t20\tFF\tFF\tFF\tFF\tFF\tFF\r\n       303  0CF102A7   00000004    8        30\t75\tE0\t2E\t80\tFF\tFF\tFD\r\n       303  0CF101A7   00000004    8        68\t00\t97\tCC\t00\t15\t39\t29\r\n       302  1FFFFFFF   00000004    8        00\t00\tFF\tFF\tFF\tFF\tFF\tFF\r\n       293  18F106A7   00000004    8        00\tF7\tFF\tFF\tFF\tFF\tFF\t76\r\n       343  0CF101A7   00000004    8        68\t00\t97\tCC\t00\t15\t39\t2B\r\n       342  18F120F0   00000004    8        2B\t75\t60\tB1\tB0\t01\tFF\tFF\r\n       341  18F11FF0   00000004    8        FF\t3F\t90\t68\t88\t1B\t10\tBC\r\n       332  1FFFFFFF   00000004    8        00\t00\tFF\tFF\tFF\tFF\tFF\tFF\r\n       323  0CF102A7   00000004    8        30\t75\tE0\t2E\t80\tFF\tFF\tFD\r\n       323  0CF101A7   00000004    8        68\t00\t97\tCC\t00\t15\t39\t2A\r\n       322  1FFFFFFF   00000004    8        00\t20\tFF\tFF\tFF\tFF\tFF\tFF\r\n       312  1FFFFFFF   00000004    8        00\t20\tFF\tFF\tFF\tFF\tFF\tFF\r\n       303  0CF102A7   00000004    8        30\t75\tE0\t2E\t80\tFF\tFF\tFD\r\n       303  0CF101A7   00000004    8        68\t00\t97\tCC\t00\t15\t39\t29\r\n       302  1FFFFFFF   00000004    8        00\t00\tFF\tFF\tFF\tFF\tFF\tFF\r\n       343  0C3C4D4A   00000004    8        BE\tFF\tFF\t7F\t18\tFF\tFF\t3B\r\n       343  0CF101A7   00000004    8        68\t00\t97\tCC\t00\t15\t39\t2B\r\n       342  18F120F0   00000004    8        2B\t75\t60\tB1\tB0\t01\tFF\tFF\r\n       341  18F11FF0   00000004    8        FF\t3F\t90\t68\t88\t1B\t10\tBC\r\n       332  1FFFFFFF   00000004    8        00\t00\tFF\tFF\tFF\tFF\tFF\tFF\r\n       323  0CF102A7   00000004    8        30\t75\tE0\t2E\t80\tFF\tFF\tFD\r\n       323  0CF101A7   00000004    8        68\t00\t97\tCC\t00\t15\t39\t2A\r\n       322  1FFFFFFF   00000004    8        00\t20\tFF\tFF\tFF\tFF\tFF\tFF\r\n       312  1FFFFFFF   00000004    8        00\t20\tFF\tFF\tFF\tFF\tFF\tFF\r\n       303  0CF102A7   00000004    8        30\t75\tE0\t2E\t80\tFF\tFF\tFD\r\n       303  0CF101A7   00000004    8        68\t00\t97\tCC\t00\t15\t39\t29\r\n       344  0CF102A7   00000004    8        30\t75\tE0\t2E\t80\tFF\tFF\tFD\r\n       343  0C3C4D4A   00000004    8        BE\tFF\tFF\t7F\t18\tFF\tFF\t3B\r\n       343  0CF101A7   00000004    
